vi "SR Type Sort.vi"(11 "list in":T1[](array[typedef]) {"Creation Date" format="%<%x>T"; "Last Updated" format="%<%x>T"}) -> (3 "Array":T1[](array[typedef]) {"Creation Date" format="%<%x>T"; "Last Updated" format="%<%x>T"})   [LabVIEW 2018]
uses:
  Type Defs/SR Cluster.ctl
  Type Defs/SR Status.ctl
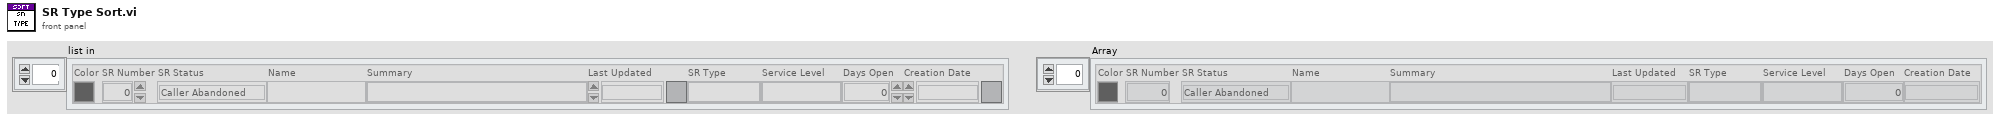
[diagram p1: front panel]
types:
  T1 = typedef "SR Cluster.ctl" = cluster{"Color":u32, "SR Number":i32, "SR Status":T2, "Name":string, "Summary":string, "Last Updated":timestamp, "SR Type":string, "Service Level":string, "Days Open":dbl, "Creation Date":timestamp}
  T2 = typedef "SR Status.ctl" = enum16{"Caller Abandoned", "Created in Error", "Expired", "Forum Resolved AE", "Forum Resolved Customer", "IN WORK", "IN WORK Collab with AES", "IN WORK Collab with PSE", "IN WORK Collab with SE", "IN WORK Customer Added Note", "IN WORK Escalation", "IN WORK Wait on Customer", "Open", "Potentially Resolved", "Presumed Resolved", "RMA Approved for Return", "RMA Closed", "RMA Closed - DOA", "RMA In Progress", "RMA Open", "RMA Waiting on Customer", "Resolved", "Passed Off"}
  T3 = cluster{"SR Type":string, string, dbl, dbl, "SR Cluster":T1}
  T4 = cluster{"SR Type":string, string, dbl, dbl, "SR Cluster":T1}[]
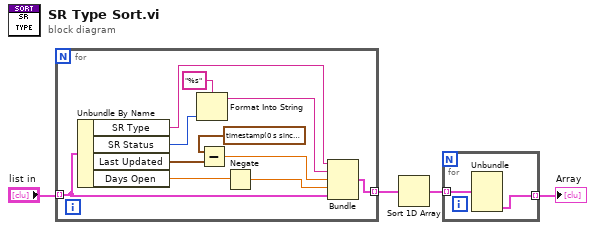
[diagram p0: block diagram]
diagram:
  n1 = for {
    tunnel: "list in" -> [w8] mode=indexing
    tunnel: [w15] -> w1 mode=indexing
    n2 = Unbundle By Name(w8) -> ("SR Type"=w5:string, "SR Status"=w14:T2, "Last Updated"=w9:timestamp, "Days Open"=w7:dbl)
    n3 = Format Into String(format string="%s", w14) -> (resulting string=w11:string)  [unwired: 2 in, 1 out]
    n4 = Subtract(x=timestamp(0 s since 1904-01-01), y=w9) -> (x-y=w10:dbl)
    n5 = Negate(x=w7) -> (-x=w6:dbl)
    n6 = Bundle("SR Type"=w5, w11, w10, w6, "SR Cluster"=w8) -> (w15:T3)  [unwired: 1 in]
  }
  n7 = Sort 1D Array(array=w1) -> (sorted array=w2:T4)
  n8 = for {
    tunnel: w2 -> [w17] mode=indexing
    tunnel: [w16] -> w4 mode=indexing
    n9 = Unbundle(w17) -> ("SR Cluster"=w16:T1)  [unwired: 4 out]
  }
  "Array" <- w4
